vi "LSX Get Stop Polarity.vi"(8 "error in (no error)":errorcluster, 10 "pbHighActiv":i32, 11 "lLSID":i32) -> (0 "error out":errorcluster, 2 "pbHighActiv out":i32, 3 "function return":i32)   [LabVIEW 2018, in "Tango.lvlib"]
doc: "TANGOAPI int TANGOCALL LSX_GetStopPolarity (int lLSID, BOOL *pbHighActiv);"
uses:
  Tango.lvlib
  SubVIs/Tango_DLL.dll
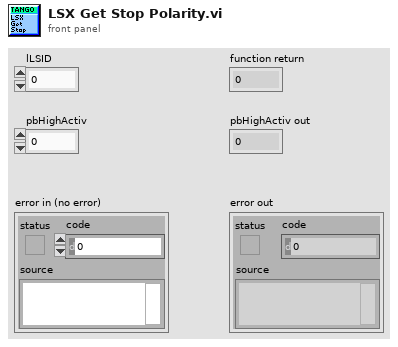
[diagram p1: front panel]
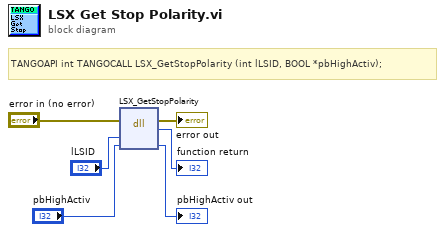
[diagram p0: block diagram]
diagram:
  # "TANGOAPI int TANGOCALL LSX_GetStopPolarity (int lLSID, BOOL *pbHighActiv);"
  n1 = dll-call lib="C:/Users/Familie/Documents/LabviewIX81/lib/TANGO Stage/SubVIs/Tango_DLL.*" fn="LSX_GetStopPolarity"(error in="error in (no error)", "lLSID"="lLSID", "pbHighActiv"="pbHighActiv") -> (error out=→"error out":errorcluster, →"function return":i32, "pbHighActiv"=→"pbHighActiv out":i32)  [unwired: 3 in, 1 out]
